vi "test.numeric_conversion.vi"   [LabVIEW 2020]
uses:
  43c55db3-e9fc-4819-8629-a2ea7ebd1e83.vi
  6755348f-4a37-4a7b-9aa8-f0de1a538cec.vi
  8c764fbb-a14c-4fea-9625-2b809bd1a02f.vi
  <vilib>/addons/_JKI Toolkits/Caraya/classes/Assert/Assert Equal Value_Variant.vi
  <vilib>/addons/_JKI Toolkits/Caraya/classes/Assert/Assert Equal Value and Type_Variant.vi
  <vilib>/addons/_JKI Toolkits/Caraya/classes/Test/Test.lvclass
  configuration-data/configuration-data.lvclass
  <vilib>/addons/_JKI Toolkits/Caraya/classes/Assert/Assert.lvclass
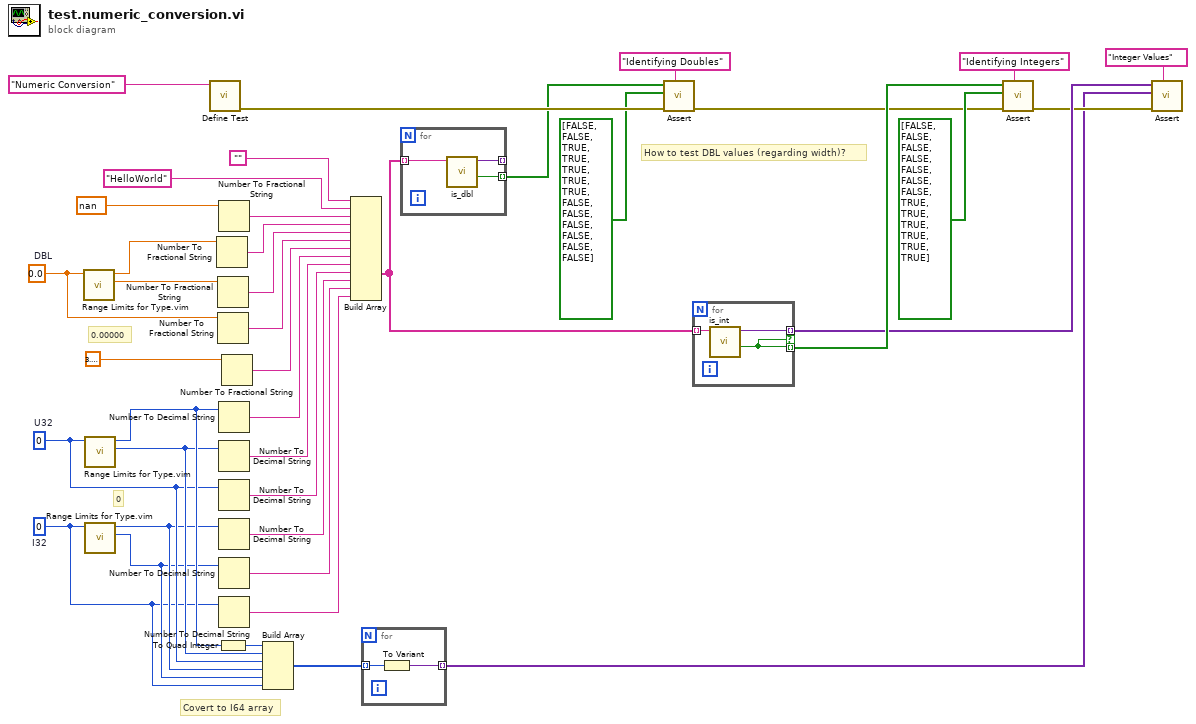
[diagram p0: block diagram]
diagram:
  w32 = 0.0  # DBL
  w7 = 0  # I32
  w10 = u32 0  # U32
  # "How to test DBL values (regarding width)?"
  # "Covert to I64 array"
  # "0"
  # "0.00000"
  n1 = call "Range Limits for Type.vim"("type"=w32) -> ("minimum value for type"=w31:dbl, "maximum value for type"=w30:dbl)  [unwired: 9 in]
  n2 = call "Range Limits for Type.vim"("type"=w10) -> ("minimum value for type"=w11:u32, "maximum value for type"=w12:u32)  [unwired: 9 in]
  n3 = call "Range Limits for Type.vim"("type"=w7) -> ("minimum value for type"=w8:i32, "maximum value for type"=w9:i32)  [unwired: 9 in]
  n4 = call <vilib>:"Define Test.vi"("Label (VI Title)"="Numeric Conversion") -> ("error out"=w21:errorcluster)  [unwired: 10 in]
  n5 = Number To Fractional String(number=w30) -> (F-format string=w27:string)  [unwired: 3 in]
  n6 = Number To Fractional String(number=w31) -> (F-format string=w28:string)  [unwired: 3 in]
  n7 = Number To Fractional String(number=w32) -> (F-format string=w29:string)  [unwired: 3 in]
  n8 = To Quad Integer(1:w12) -> (0:w2:i64)
  n9 = Number To Fractional String(number=nan) -> (F-format string=w26:string)  [unwired: 3 in]
  n10 = Number To Decimal String(number=w12) -> (decimal integer string=w39:string)  [unwired: 1 in]
  n11 = Number To Decimal String(number=w11) -> (decimal integer string=w38:string)  [unwired: 1 in]
  n12 = Number To Decimal String(number=w10) -> (decimal integer string=w37:string)  [unwired: 1 in]
  n13 = Number To Decimal String(number=w9) -> (decimal integer string=w36:string)  [unwired: 1 in]
  n14 = Number To Decimal String(number=w8) -> (decimal integer string=w35:string)  [unwired: 1 in]
  n15 = Number To Decimal String(number=w7) -> (decimal integer string=w34:string)  [unwired: 1 in]
  n16 = Number To Fractional String(number=3.141592653589793) -> (F-format string=w24:string)  [unwired: 3 in]
  n17 = Build Array(w2, w11, w10, w9, w8, w7) -> (w1:i64[])
  n18 = Build Array("", "HelloWorld", w26, w27, w28, w29, w24, w39, w38, w37, w36, w35, w34) -> (w13:string[])
  n19 = for {
    tunnel: w1 -> [w42] mode=indexing
    tunnel: [w41] -> w3 mode=indexing
    n20 = To Variant(anything=w42) -> (Variant=w41:variant)
  }
  n21 = for {
    tunnel: w13 -> [w45] mode=indexing
    tunnel: [w44] -> w19 mode=indexing
    tunnel: [w43] -> _ mode=indexing
    n22 = call "is_dbl.vi"("data in"=w45) -> ("confirmed?"=w44:bool, "data out"=w43:variant)  [unwired: 9 in]
  }
  n23 = call-poly <vilib>:"Assert.vi"("Label"="Identifying Doubles", "error in (no error)"=w21, "Y"=bool[] [FALSE, FALSE, TRUE, TRUE, TRUE, TRUE, TRUE, FALSE, FALSE, FALSE, FALSE, FALSE, FALSE] ("Array 2"), "X"=w19) -> ("error out"=w14:errorcluster)  [unwired: 7 in]
  n24 = for {
    tunnel: [w47] -> w16 mode=indexing
    tunnel: w13 -> [w48] mode=indexing
    tunnel: [w46] -> w6 mode=indexing if=w47
    n25 = call "is_int.vi"("data in"=w48) -> ("confirmed?"=w47:bool, "data out"=w46:variant)  [unwired: 9 in]
  }
  n26 = call-poly <vilib>:"Assert.vi"("Label"="Identifying Integers", "error in (no error)"=w14, "Y"=bool[] [FALSE, FALSE, FALSE, FALSE, FALSE, FALSE, FALSE, TRUE, TRUE, TRUE, TRUE, TRUE, TRUE] ("Array 2"), "X"=w16) -> ("error out"=w4:errorcluster)  [unwired: 7 in]
  n27 = call-poly <vilib>:"Assert.vi"("Label"="Integer Values", "error in (no error)"=w4, "Y"=w3, "X"=w6) -> ()  [unwired: 7 in, 1 out]
